vi "グラフ確認.vi"() -> ()   [LabVIEW 2016]
uses:
  <vilib>/measure/NI_MABase.lvlib
  <vilib>/measure/NI_MAPro.lvlib
panel:
  in  "停止":bool
  out "波形グラフ(波形)":waveform(dbl)[](graph)
  out "XYグラフ(DBL)":cluster{"Y":dbl[], "Y":dbl[]}(graph)
  out "波形グラフ(DBL)":cluster{"X0":dbl, "dt":dbl, "Y":dbl[]}[](graph)
  out "波形チャート":dbl[][](graph)
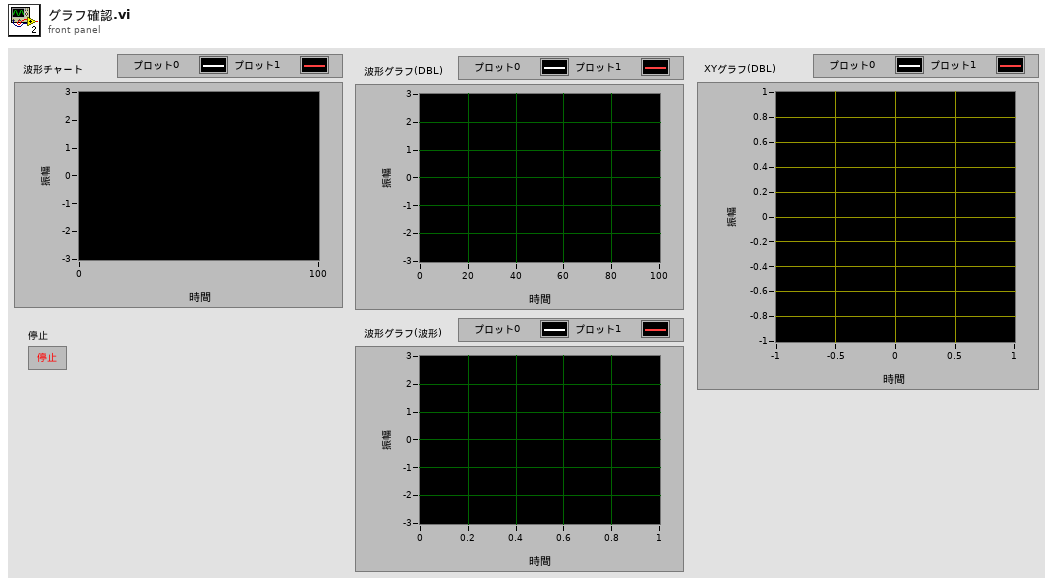
[diagram p1: front panel]
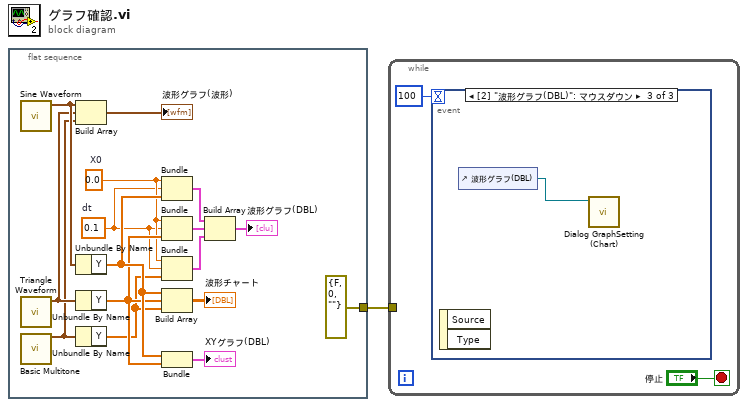
[diagram p0: block diagram]
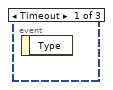
[diagram p2: hidden frame]
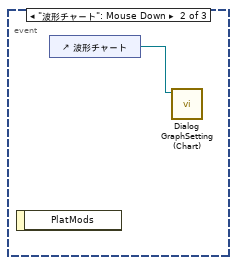
[diagram p3: hidden frame]
diagram:
  n1 = flat-sequence {
    tunnel: [errorcluster {"status"=FALSE, "code"=0, "source"=""} ("エラー定数")] -> w1
    frame #0 {
      w7 = 0.1  # dt
      w8 = 0.0  # X0
      n2 = call <vilib>:"Sine Waveform.vi"() -> ("signal out"=w13:waveform(dbl))  [unwired: 10 in, 1 out]
      n3 = call <vilib>:"Triangle Waveform.vi"() -> ("signal out"=w12:waveform(dbl))  [unwired: 10 in, 1 out]
      n4 = call <vilib>:"Basic Multitone.vi"() -> ("signal out"=w4:waveform(dbl))  [unwired: 12 in, 3 out]
      n5 = Build Array(w13, w12, w4) -> (→"波形グラフ(波形)":waveform(dbl)[])
      n6 = Unbundle By Name(w13) -> ("Y"=w11:dbl[])
      n7 = Unbundle By Name(w12) -> ("Y"=w10:dbl[])
      n8 = Unbundle By Name(w4) -> ("Y"=w6:dbl[])
      n9 = Bundle("X0"=w8, "dt"=w7, "Y"=w11) -> (w16:cluster{"X0":dbl, "dt":dbl, "Y":dbl[]})  [unwired: 1 in]
      n10 = Bundle("X0"=w8, "dt"=w7, "Y"=w10) -> (w15:cluster{"X0":dbl, "dt":dbl, "Y":dbl[]})  [unwired: 1 in]
      n11 = Bundle("X0"=w8, "dt"=w7, "Y"=w6) -> (w5:cluster{"X0":dbl, "dt":dbl, "Y":dbl[]})  [unwired: 1 in]
      n12 = Build Array(w11, w10, w6) -> (→"波形チャート":dbl[][])
      n13 = Bundle("Y"=w11, "Y"=w10) -> (→"XYグラフ(DBL)":cluster{"Y":dbl[], "Y":dbl[]})  [unwired: 1 in]
      n14 = Build Array(w16, w15, w5) -> (→"波形グラフ(DBL)":cluster{"X0":dbl, "dt":dbl, "Y":dbl[]}[])
    }
  }
  n15 = while {
    tunnel: w1 -> [_]
    stop <- "停止" stop-if-true
    n16 = event shown="[2] \"波形グラフ(DBL)\": マウスダウン" {
      selector: _ -> [_ _ _]
      dyn-events: _ -> [_ _ _]
      timeout: 100 -> [_ _ _]
      event Timeout {
        n17 = event-data() -> ()  [unwired: 1 in, 1 out]
      }
      event "波形チャート": Mouse Down {
        n18 = event-data() -> ()  [unwired: 1 in, 1 out]
        n19 = control-ref of="波形チャート"() -> (w20:refnum<vi>)
        n20 = call "Dialog GraphSetting (Chart).vi"("波形チャートref(in)"=w20) -> ()  [unwired: 11 in]
      }
      event "波形グラフ(DBL)": Mouse Down {
        n21 = event-data() -> ()  [unwired: 1 in, 2 out]
        n22 = control-ref of="波形グラフ(DBL)"() -> (w21:refnum<vi>)
        n23 = call "Dialog GraphSetting (Chart).vi"("波形チャートref(in)"=w21) -> ()  [unwired: 11 in]
      }
    }
  }
